vi "StageUpdate.vi"(0 "Microscope in":refnum<class "Microscope.lvclass">, 7 "Stage events":refnum<queue>, 9 "X Data":refnum<queue>, 11 "error in (no error)":errorcluster) -> (4 "Microscope out":refnum<class "Microscope.lvclass">, 8 "Image full":bool, 10 "stop loop":bool, 15 "error out":errorcluster)   [LabVIEW 2012, in "Microscope.lvclass"]
uses:
  classes/Microscope.lvclass
  typedefs/StageEvent.ctl
  classes/Microscope.lvclass/Microscope.ctl
  typedefs/Move Type.ctl
  variables/GlobalUI.vi
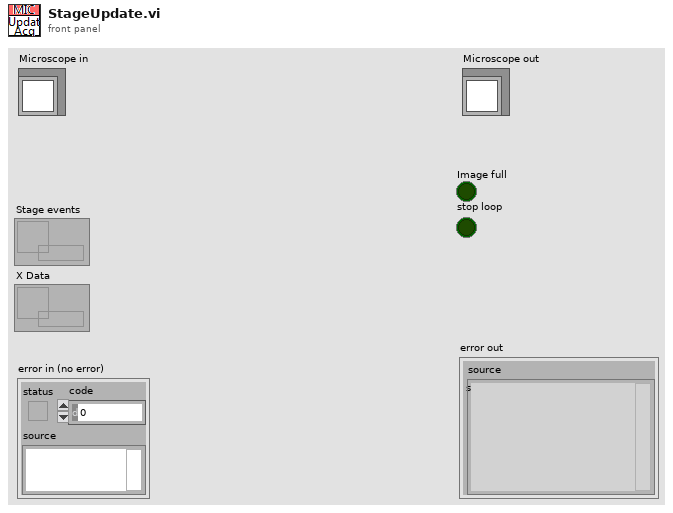
[diagram p1: front panel]
types:
  T1 = typedef "DetectorType.ctl" = enum16{"PMT", "SpectraWiz"}
  T2 = typedef "Move Type.ctl" = enum16{"None", "Continuous", "Discrete"}
  T3 = typedef "StageEvent.ctl" = enum16{"stage.TimeOut", "stage.FlushData", "stage.GetPosition", "stage.Init", "stage.MoveTo1", "stage.MoveTo2", "stage.MoveTo3", "stage.Stop"}
  T4 = typedef "ScanMode.ctl" = enum16{"None", "Continuous", "Point Scan (CH3 cursor)", "Point Scan Move (CH3 cursor)", "Grab", "Grab Move Stage", "Grab Move Z-stage", "Cont. Move Z-stage", "Spec Move Stage", "Spec Move Cont", "Surf Calib"}
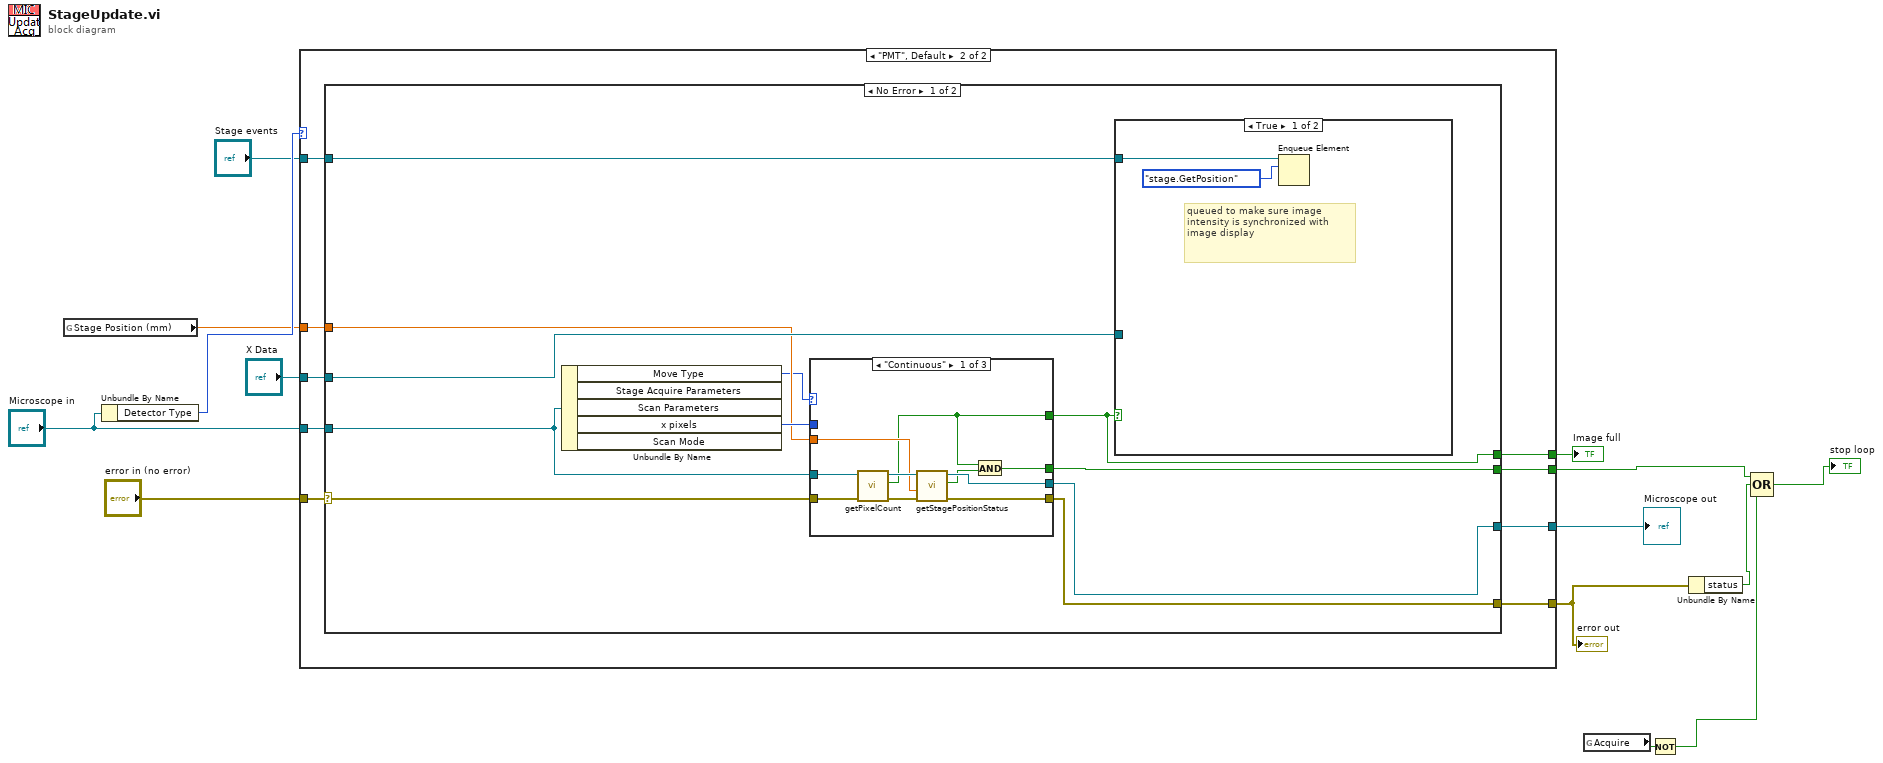
[diagram p0: block diagram]
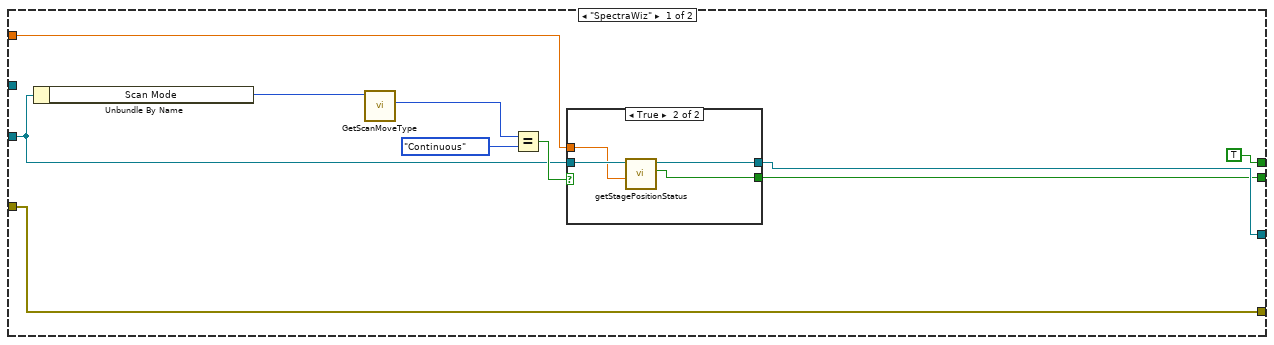
[diagram p2: hidden frame]
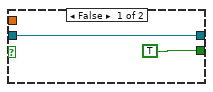
[diagram p3: hidden frame]
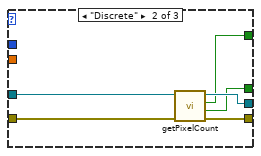
[diagram p5: hidden frame]
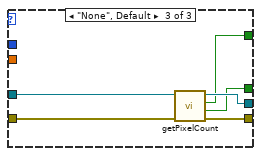
[diagram p6: hidden frame]
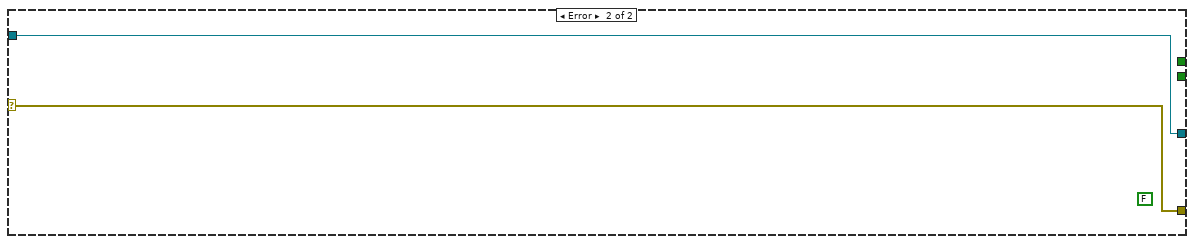
[diagram p7: hidden frame]
diagram:
  n1 = global read "GlobalUI.vi" "Stage Position (mm)"() -> (w9:dbl)
  n2 = Unbundle By Name("Microscope in") -> ("Detector Type"=w10:T1)
  n3 = case shown="\"PMT\", Default" w10 {
    tunnel: "error in (no error)" -> [w24 w39]
    tunnel: [w24 w38] -> w6
    tunnel: [w18 w37] -> w13
    tunnel: [w16 w36] -> w5
    tunnel: w9 -> [w17 w35]
    tunnel: "X Data" -> [_ w34]
    tunnel: "Microscope in" -> [w19 w33]
    tunnel: [TRUE ("Image full") w32] -> w8
    tunnel: "Stage events" -> [_ w31]
    frame "SpectraWiz" {
      n4 = Unbundle By Name(w19) -> ("Scan Mode"=w23:T4)
      n5 = call "GetScanMoveType.vi"("Scan Mode"=w23) -> ("Move Type"=w22:T2)  [unwired: 8 in, 2 out]
      n6 = Equal?(x=w22, y=Move_Type."Continuous") -> (x = y?=w20:bool)
      n7 = case shown="True" w20 {
        tunnel: w19 -> [w26 w30]
        tunnel: [w26 w29] -> w18
        tunnel: w17 -> [_ w28]
        tunnel: [TRUE ("Grabbed all required frames?") w27] -> w16
        frame False {
        }
        frame True {
          n8 = call "getStagePositionStatus.vi"("Stage Position (mm)"=w28, "Microscope in"=w30) -> ("stage position ok"=w27:bool, "Microscope out"=w29:refnum<class "Microscope.lvclass">)  [unwired: 7 in, 1 out]
        }
      }
    }
    frame "PMT", Default {
      n9 = case shown="No Error" w39 {
        selector: w39 -> [w46 w76]
        tunnel: [w47 w76] -> w38
        tunnel: [w50 w75] -> w37
        tunnel: w33 -> [w48 w75]
        tunnel: [w42 _] -> w36
        tunnel: w35 -> [w44 _]
        tunnel: w34 -> [w45 _]
        tunnel: [w41 _] -> w32
        tunnel: w31 -> [w40 _]
        frame No Error {
          n10 = Unbundle By Name(w48) -> ("Move Type"=w43:T2, "x pixels"=w49:i32)  [unwired: 3 out]
          n11 = case shown="\"Continuous\"" w43 {
            tunnel: [w53 w63 w69] -> w42
            tunnel: [w61 w67 w73] -> w50
            tunnel: w49 -> [_ _ _]
            tunnel: w48 -> [w60 w68 w74]
            tunnel: [w62 w66 w72] -> w47
            tunnel: w46 -> [w58 w65 w71]
            tunnel: w44 -> [w56 _ _]
            tunnel: [w55 w64 w70] -> w41
            frame "Continuous" {
              n12 = call "getPixelCount.vi"("error in (no error)"=w58, "Microscope in"=w60) -> ("error out"=w57:errorcluster, "Image full"=w55:bool, "Microscope out"=w59:refnum<class "Microscope.lvclass">)  [unwired: 6 in, 1 out]
              n13 = call "getStagePositionStatus.vi"("error in (no error)"=w57, "Stage Position (mm)"=w56, "Microscope in"=w59) -> ("error out"=w62:errorcluster, "stage position ok"=w54:bool, "Microscope out"=w61:refnum<class "Microscope.lvclass">)  [unwired: 6 in]
              n14 = And(x=w55, y=w54) -> (x .and. y?=w53:bool)
            }
            frame "Discrete" {
              n15 = call "getPixelCount.vi"("error in (no error)"=w65, "Microscope in"=w68) -> ("error out"=w66:errorcluster, "Grabbed all required frames?"=w63:bool, "Image full"=w64:bool, "Microscope out"=w67:refnum<class "Microscope.lvclass">)  [unwired: 6 in]
            }
            frame "None", Default {
              n16 = call "getPixelCount.vi"("error in (no error)"=w71, "Microscope in"=w74) -> ("error out"=w72:errorcluster, "Grabbed all required frames?"=w69:bool, "Image full"=w70:bool, "Microscope out"=w73:refnum<class "Microscope.lvclass">)  [unwired: 6 in]
            }
          }
          n17 = case shown="True" w41 {
            tunnel: w45 -> [_ _]
            tunnel: w40 -> [w51 _]
            frame True {
              # "queued to make sure image intensity is synchronized with image display"
              n18 = Enqueue Element(queue=w51, element=StageEvent."stage.GetPosition") -> ()  [unwired: 2 in, 3 out]
            }
            frame False {
            }
          }
        }
        frame Error {
          (unwired) FALSE ("bWait")
        }
      }
    }
  }
  "error out" <- w6
  "Microscope out" <- w13
  "Image full" <- w8
  n19 = global read "GlobalUI.vi" "Acquire"() -> (w1:bool)
  n20 = Not(x=w1) -> (.not. x?=w2:bool)
  n21 = Unbundle By Name(w6) -> ("status"=w4:bool)
  n22 = Compound Arithmetic op=OR(w5, w4, w2) -> (→"stop loop":bool)
